vi "Teleop.vi"(10 "Match Info":T1={"Autonomous Elapsed Seconds"=0.0, "TeleOp Elapsed Seconds"=0.0, "Disabled Elapsed Seconds"=0.0, "Visited Autonomous"=FALSE, "Visited TeleOp"=FALSE, "Visited Disabled"=FALSE, "Autonomous Settings"={"Autonomous Style"=enum."Independent", "VI Refnum"=refnum}}, 11 "Call Context":T2) -> ()   [LabVIEW 2020]
doc: "This VI is called for each TeleOp packet received from the DS where the robot is not disabled. It is often used to read from the joysticks and update I/O or to update setpoints for timed control loops. It should complete and return within 20 milliseconds or it may miss DS packets."
uses:
  <vilib>/Rock Robotics/WPI/DriverStation/WPI_DriverStationDerivedRobotMode.ctl
  <vilib>/Rock Robotics/WPI/DriverStation/WPI_DriverStationMatch Info.ctl
  <vilib>/Rock Robotics/WPI/Utilities/WPI_GetSetVariantRefNum.vi
  Global Variables/Axes_N_Buttons.vi
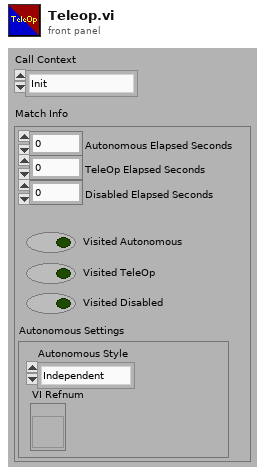
[diagram p1: front panel]
types:
  T1 = typedef "WPI_DriverStationMatch Info.ctl" = cluster{"Autonomous Elapsed Seconds":dbl, "TeleOp Elapsed Seconds":dbl, "Disabled Elapsed Seconds":dbl, "Visited Autonomous":bool, "Visited TeleOp":bool, "Visited Disabled":bool, "Autonomous Settings":cluster{"Autonomous Style":enum16{"Iterative", "Independent"}, "VI Refnum":refnum<vi>}}
  T2 = typedef "WPI_DriverStationDerivedRobotMode.ctl" = enum16{"Init", "Execute", "Stop"}
  T3 = typedef "WPI_JoystickDevRef.ctl" = cluster{"Device":T4}
  T4 = typedef "WPI_JoystickDeviceEnum.ctl" = enum16{"USB 0", "USB 1", "USB 2", "USB 3", "USB 4", "USB 5"}
  T5 = typedef "Button Cluster.ctl" = cluster{"Buttons[0]":bool, "Buttons[1]":bool, "Buttons[2]":bool, "Buttons[3]":bool, "Buttons[4]":bool, "Buttons[5]":bool, "Buttons[6]":bool, "Buttons[7]":bool, "Buttons[8]":bool, "Buttons[9]":bool}
  T6 = typedef "Axes Cluster.ctl" = cluster{"Axes[0]":dbl, "Axes[1]":dbl, "Axes[2]":dbl, "Axes[3]":dbl, "Axes[4]":dbl, "Axes[5]":dbl, "Axes[6]":dbl, "Axes[7]":dbl, "Axes[8]":dbl}
  T7 = typedef "D-Pad.ctl" = cluster{"Top":bool, "Bottom":bool, "None":bool, "Right":bool, "Left":bool}
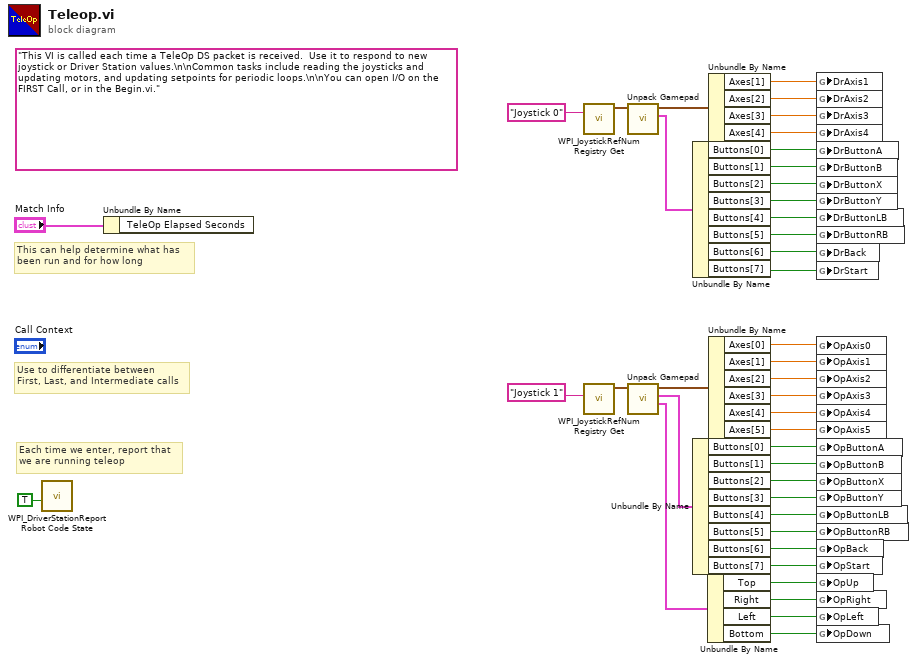
[diagram p0: block diagram]
diagram:
  (unwired) "This VI is called each time a TeleOp DS packet is received.  Use it to respond to new joystick or Driver Station values.\n\nCommon tasks include reading the joysticks and updating motors, and updating setpoints for periodic loops.\n\nYou can open I/O on the FIRST Call, or in the Begin.vi."
  # "Each time we enter, report that\nwe are running teleop"
  # "Use to differentiate between\nFirst, Last, and Intermediate calls"
  # "This can help determine what has\nbeen run and for how long"
  n1 = call <vilib>:"WPI_DriverStationReport Robot Code State.vi"("TeleOp"=TRUE ("Autonomous")) -> ()  [unwired: 10 in, 1 out]
  n2 = Unbundle By Name("Match Info") -> ()  [unwired: 1 out]
  n3 = call <vilib>:"WPI_JoystickRefNum Registry Get.vi"("refnum name"="Joystick 0") -> ("JoystickDevRef"=w37:T3)  [unwired: 1 in, 9 out]
  n4 = call <vilib>:"WPI_JoystickRefNum Registry Get.vi"("refnum name"="Joystick 1") -> ("JoystickDevRef"=w36:T3)  [unwired: 1 in, 9 out]
  n5 = call "Unpack Gamepad.vi"("JoystickDevRef"=w37) -> ("Button Cluster"=w29:T5, "Axes"=w34:T6)  [unwired: 8 in, 1 out]
  n6 = call "Unpack Gamepad.vi"("JoystickDevRef"=w36) -> ("D-Pad"=w7:T7, "Button Cluster"=w16:T5, "Axes"=w35:T6)  [unwired: 8 in]
  n7 = Unbundle By Name(w29) -> ("Buttons[0]"=w28:bool, "Buttons[1]"=w27:bool, "Buttons[2]"=w26:bool, "Buttons[3]"=w25:bool, "Buttons[4]"=w24:bool, "Buttons[5]"=w23:bool, "Buttons[6]"=w2:bool, "Buttons[7]"=w1:bool)
  n8 = Unbundle By Name(w16) -> ("Buttons[0]"=w15:bool, "Buttons[1]"=w14:bool, "Buttons[2]"=w13:bool, "Buttons[3]"=w12:bool, "Buttons[4]"=w11:bool, "Buttons[5]"=w10:bool, "Buttons[6]"=w9:bool, "Buttons[7]"=w8:bool)
  n9 = Unbundle By Name(w7) -> ("Top"=w6:bool, "Right"=w5:bool, "Left"=w4:bool, "Bottom"=w3:bool)
  n10 = Unbundle By Name(w34) -> ("Axes[1]"=w33:dbl, "Axes[2]"=w32:dbl, "Axes[3]"=w31:dbl, "Axes[4]"=w30:dbl)
  n11 = Unbundle By Name(w35) -> ("Axes[0]"=w22:dbl, "Axes[1]"=w21:dbl, "Axes[2]"=w20:dbl, "Axes[3]"=w19:dbl, "Axes[4]"=w18:dbl, "Axes[5]"=w17:dbl)
  n12 = global write "Axes_N_Buttons.vi" "DrAxis1"(w33) -> ()
  n13 = global write "Axes_N_Buttons.vi" "DrAxis2"(w32) -> ()
  n14 = global write "Axes_N_Buttons.vi" "DrAxis3"(w31) -> ()
  n15 = global write "Axes_N_Buttons.vi" "DrAxis4"(w30) -> ()
  n16 = global write "Axes_N_Buttons.vi" "DrButtonA"(w28) -> ()
  n17 = global write "Axes_N_Buttons.vi" "DrButtonB"(w27) -> ()
  n18 = global write "Axes_N_Buttons.vi" "DrButtonX"(w26) -> ()
  n19 = global write "Axes_N_Buttons.vi" "DrButtonY"(w25) -> ()
  n20 = global write "Axes_N_Buttons.vi" "DrButtonLB"(w24) -> ()
  n21 = global write "Axes_N_Buttons.vi" "DrButtonRB"(w23) -> ()
  n22 = global write "Axes_N_Buttons.vi" "DrBack"(w2) -> ()
  n23 = global write "Axes_N_Buttons.vi" "DrStart"(w1) -> ()
  n24 = global write "Axes_N_Buttons.vi" "OpAxis0"(w22) -> ()
  n25 = global write "Axes_N_Buttons.vi" "OpAxis1"(w21) -> ()
  n26 = global write "Axes_N_Buttons.vi" "OpAxis2"(w20) -> ()
  n27 = global write "Axes_N_Buttons.vi" "OpAxis3"(w19) -> ()
  n28 = global write "Axes_N_Buttons.vi" "OpAxis4"(w18) -> ()
  n29 = global write "Axes_N_Buttons.vi" "OpAxis5"(w17) -> ()
  n30 = global write "Axes_N_Buttons.vi" "OpButtonA"(w15) -> ()
  n31 = global write "Axes_N_Buttons.vi" "OpButtonB"(w14) -> ()
  n32 = global write "Axes_N_Buttons.vi" "OpButtonX"(w13) -> ()
  n33 = global write "Axes_N_Buttons.vi" "OpButtonY"(w12) -> ()
  n34 = global write "Axes_N_Buttons.vi" "OpButtonLB"(w11) -> ()
  n35 = global write "Axes_N_Buttons.vi" "OpButtonRB"(w10) -> ()
  n36 = global write "Axes_N_Buttons.vi" "OpBack"(w9) -> ()
  n37 = global write "Axes_N_Buttons.vi" "OpStart"(w8) -> ()
  n38 = global write "Axes_N_Buttons.vi" "OpUp"(w6) -> ()
  n39 = global write "Axes_N_Buttons.vi" "OpRight"(w5) -> ()
  n40 = global write "Axes_N_Buttons.vi" "OpLeft"(w4) -> ()
  n41 = global write "Axes_N_Buttons.vi" "OpDown"(w3) -> ()
